vi "GetPicture.vi"(8 "error in (no error)":errorcluster) -> (0 "error out":errorcluster, 3 "2D Picture":picture)   [LabVIEW 2020, in "CTI-Peripheral.lvlib" / "48x64 I2C OLED SSD1306.lvclass"]
uses:
  48x64 I2C OLED SSD1306.lvclass
  <vilib>/Utility/miscctls.llb/LVBoundsTypeDef.ctl
panel:
  # "Input"
  # "Output"
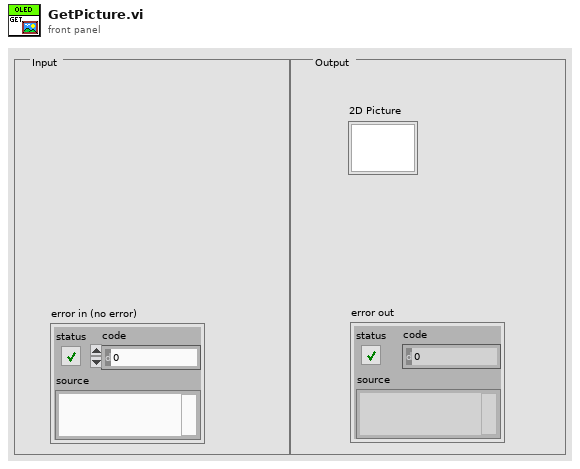
[diagram p1: front panel]
types:
  T1 = typedef "LVBoundsTypeDef.ctl" = cluster{"Width":u32, "Height":u32}
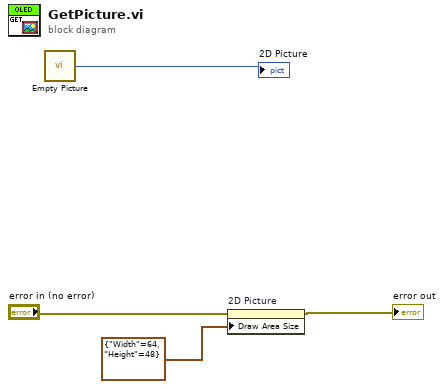
[diagram p0: block diagram]
diagram:
  n1 = call "Empty Picture"() -> ("empty picture"=→"2D Picture":picture)
  n2 = property on="2D Picture" class="Pict"(error in="error in (no error)", "Draw Area Size"=T1 {"Width"=64, "Height"=48}) -> (error out=→"error out":errorcluster)  [unwired: 1 in, 1 out]
